vi "Describe Variant.vi"(11 "Variant":variant) -> (1 "Type Description":string, 2 "Description":string, 3 "Variant Description":string)   [LabVIEW 2020, in "Comparator.lvclass"]
uses:
  Comparator.lvclass
  <vilib>/Utility/Data Type/NI_Data Type.lvlib
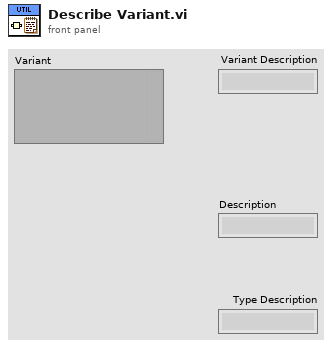
[diagram p1: front panel]
types:
  T1 = typedef "NI_Data Type.lvlib/Data Type.ctl" = enum8{"Invalid Type", "Void", "I8", "I16", "I32", "I64", "U8", "U16", "U32", "U64", "Single Float", "Double Float", "Extended Float", "Single Complex", "Double Complex", "Extended Complex", "Enum U8", "Enum U16", "Enum U32", "Enum U64", "Single Float With Unit", "Double Float With Unit", "Extended Float With Unit", "Single Complex with Unit", "Double Complex with Unit", "Extended Complex with Unit", "Boolean", "String", "Path", "Picture", "Tag", "Array", "Cluster", "Variant", "LV Variant", "Waveform", "Timestamp", "Digital Waveform", "Digital Data", "ExpressData", "Refnum", "External Data", "VI", "Poly VI", "LabVIEW Class Instance", "Fixed Point", "Set Collection", "Map Collection"}
  T2 = enum8{"Invalid Type", "Void", "I8", "I16", "I32", "I64", "U8", "U16", "U32", "U64", "Single Float", "Double Float", "Extended Float", "Single Complex", "Double Complex", "Extended Complex", "Enum U8", "Enum U16", "Enum U32", "Enum U64", "Single Float With Unit", "Double Float With Unit", "Extended Float With Unit", "Single Complex with Unit", "Double Complex with Unit", "Extended Complex with Unit", "Boolean", "String", "Path", "Picture", "Tag", "Array", "Cluster", "Variant", "LV Variant", "Waveform", "Timestamp", "Digital Waveform", "Digital Data", "ExpressData", "Refnum", "External Data", "VI", "Poly VI", "LabVIEW Class Instance", "Fixed Point", "Set Collection", "Map Collection"}
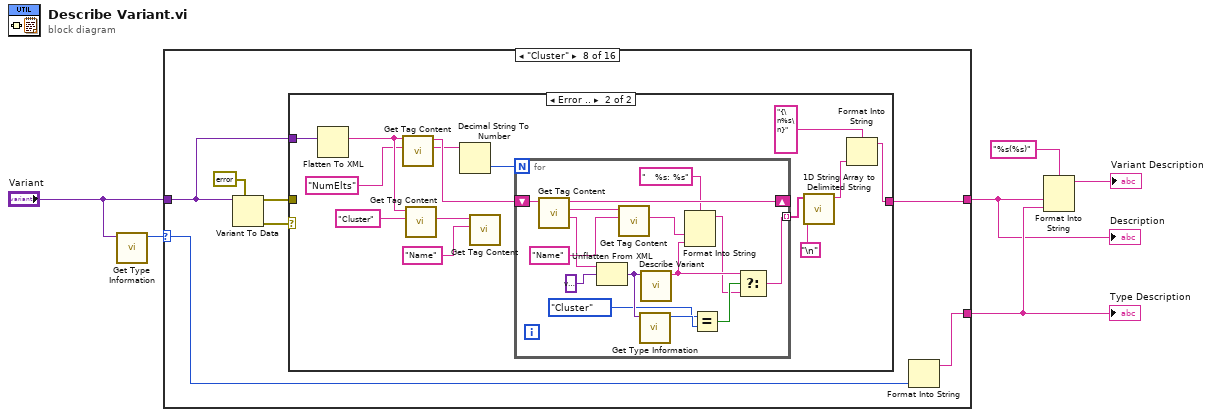
[diagram p0: block diagram]
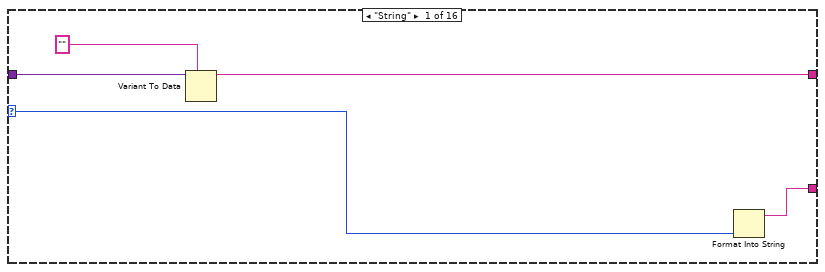
[diagram p2: hidden frame]
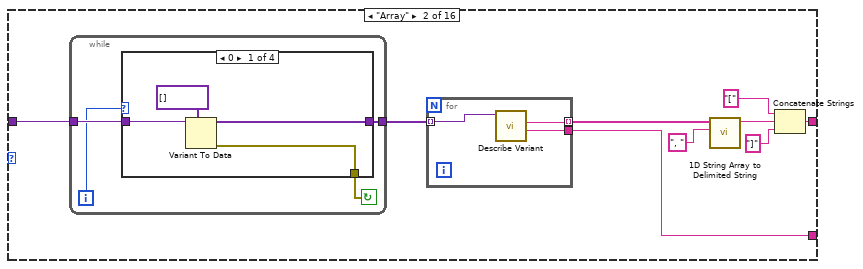
[diagram p3: hidden frame]
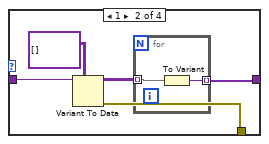
[diagram p4: hidden frame]
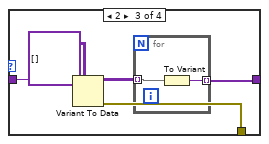
[diagram p5: hidden frame]
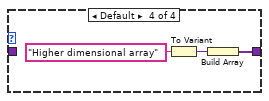
[diagram p6: hidden frame]
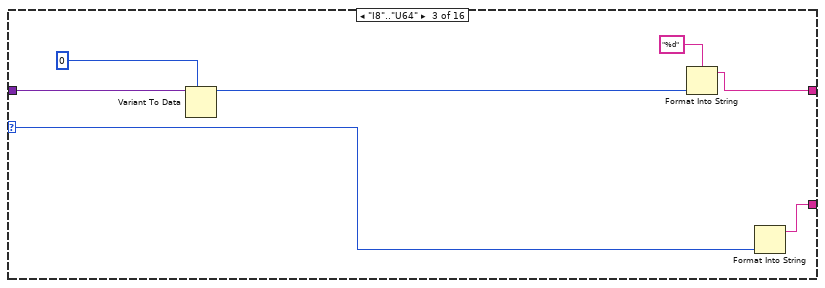
[diagram p7: hidden frame]
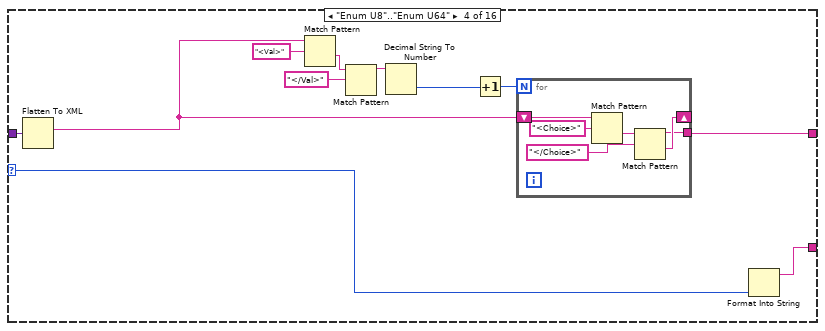
[diagram p8: hidden frame]
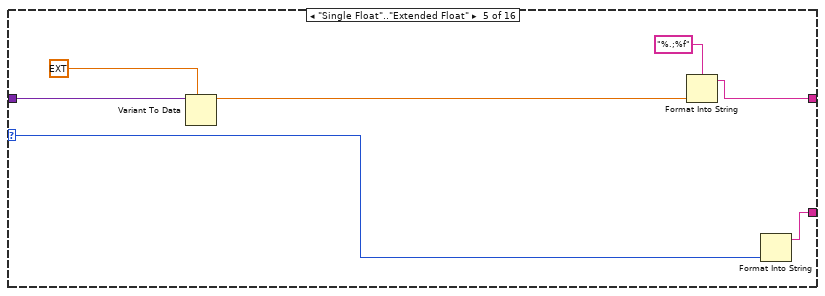
[diagram p9: hidden frame]
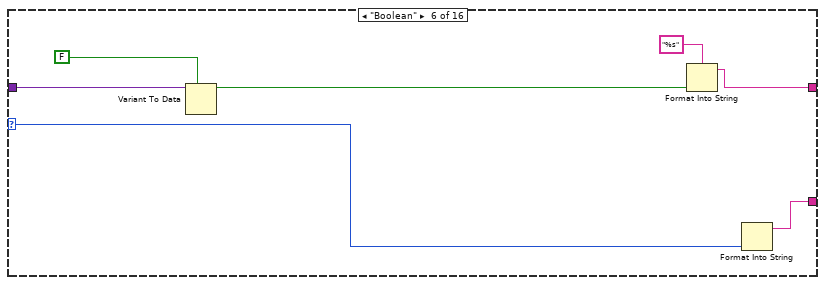
[diagram p10: hidden frame]
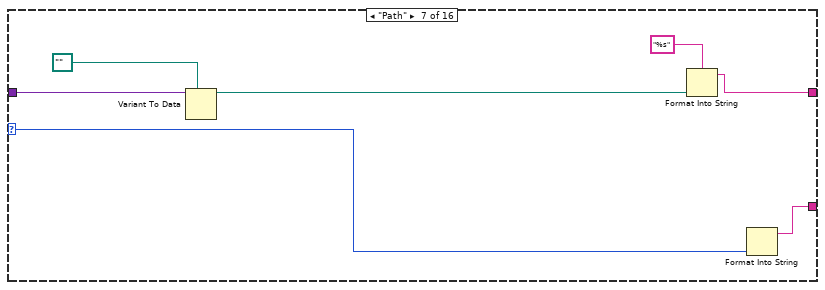
[diagram p11: hidden frame]
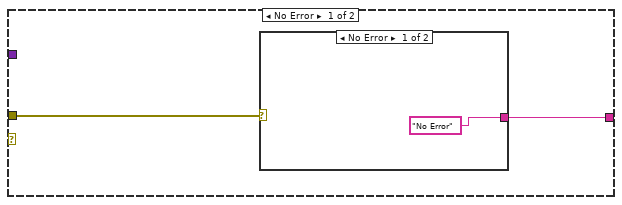
[diagram p12: hidden frame]
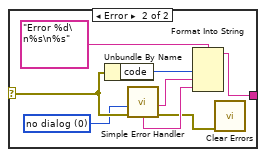
[diagram p13: hidden frame]
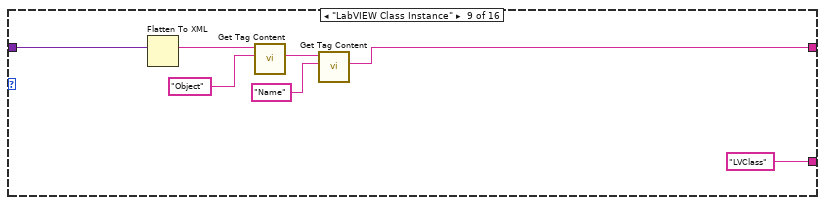
[diagram p14: hidden frame]
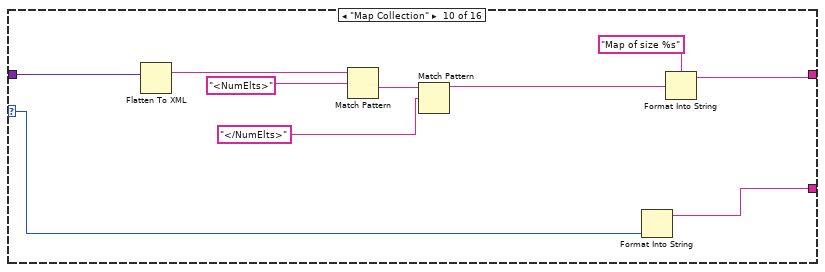
[diagram p15: hidden frame]
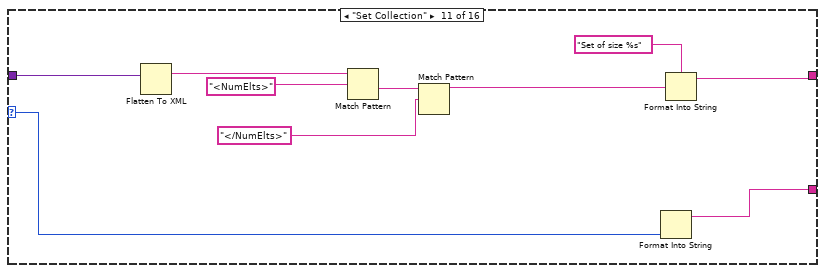
[diagram p16: hidden frame]
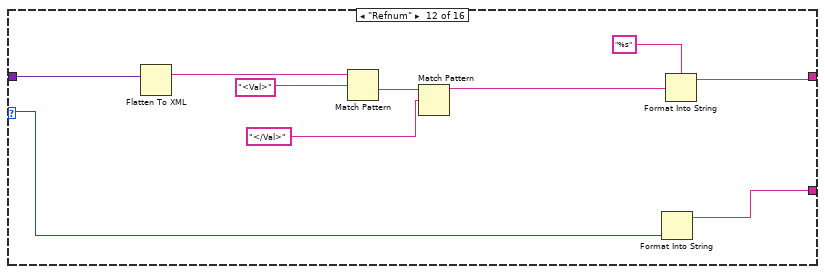
[diagram p17: hidden frame]
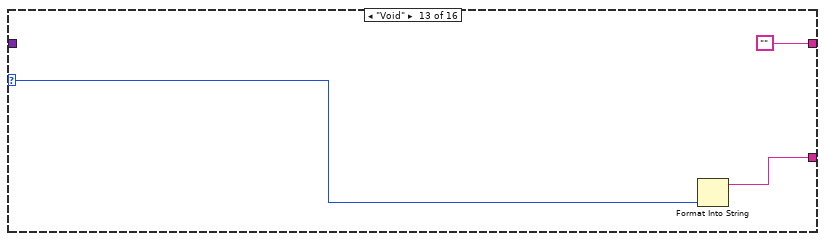
[diagram p18: hidden frame]
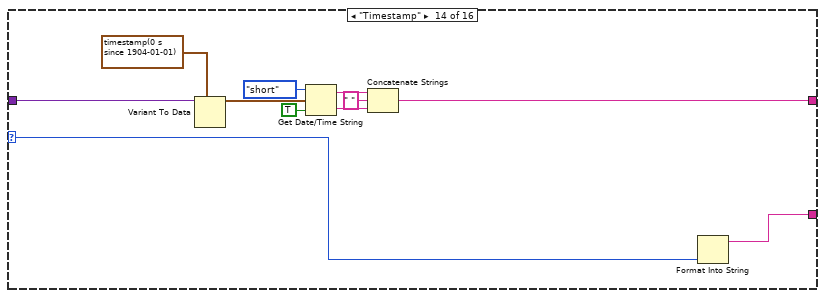
[diagram p19: hidden frame]
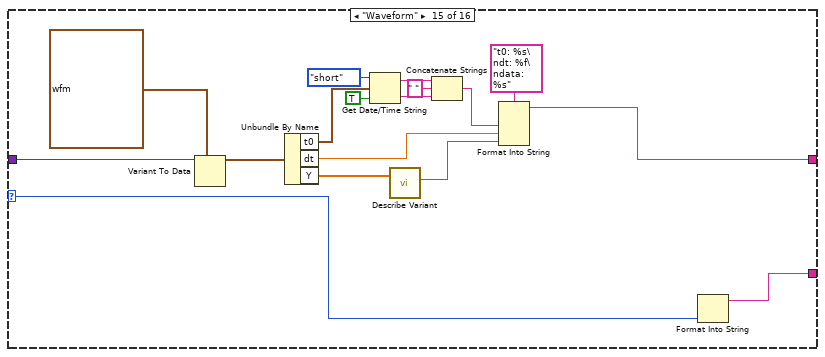
[diagram p20: hidden frame]
diagram:
  n1 = call <vilib>:"Get Type Information.vi"("variant"="Variant") -> ("type"=w5:T1)  [unwired: 6 in, 4 out]
  n2 = case shown="\"Cluster\"" w5 {
    selector: w5 -> [w7 _ w49 w65 w73 w80 w87 w98 _ w148 w158 w168 w180 w191 w208 w209]
    tunnel: "Variant" -> [w11 w20 w55 w57 w79 w86 w93 w94 w147 w157 w167 w177 _ w189 w206 w212]
    tunnel: [w10 w15 w51 w56 w75 w82 w89 w96 w141 w150 w160 w170 "" w181 w192 w211] -> w2
    tunnel: [w8 w12 w50 w66 w74 w81 w88 w97 "LVClass" w149 w159 w169 w179 w190 w207 w210] -> w4
    frame "String" {
      n3 = Variant To Data(type="", Variant=w11) -> (data=w10:string)  [unwired: 1 in, 1 out]
      n4 = Format Into String(w7) -> (resulting string=w8:string)  [unwired: 3 in, 1 out]
    }
    frame "Array" {
      n5 = while {
        tunnel: w20 -> [w24]
        tunnel: [w23] -> w19
        i -> [w22]
        stop <- w21 continue-if-true
        n6 = case shown="0" w22 {
          tunnel: w24 -> [w28 w33 w40 _]
          tunnel: [w26 w30 w37 w43] -> w23
          tunnel: [w25 w29 w36 _] -> w21
          frame 0 {
            n7 = Variant To Data(type=variant[] [], Variant=w28) -> (data=w26:variant[], error out=w25:errorcluster)  [unwired: 1 in]
          }
          frame 1 {
            n8 = Variant To Data(type=variant[][] [], Variant=w33) -> (data=w31:variant[][], error out=w29:errorcluster)  [unwired: 1 in]
            n9 = for {
              tunnel: w31 -> [w35] mode=indexing
              tunnel: [w34] -> w30 mode=indexing
              n10 = To Variant(anything=w35) -> (Variant=w34:variant)
            }
          }
          frame 2 {
            n11 = Variant To Data(type=variant[][][] [], Variant=w40) -> (data=w38:variant[][][], error out=w36:errorcluster)  [unwired: 1 in]
            n12 = for {
              tunnel: w38 -> [w42] mode=indexing
              tunnel: [w41] -> w37 mode=indexing
              n13 = To Variant(anything=w42) -> (Variant=w41:variant)
            }
          }
          frame Default {
            n14 = To Variant(anything="Higher dimensional array") -> (Variant=w44:variant)
            n15 = Build Array(w44) -> (w43:variant[])
          }
        }
      }
      n16 = for {
        tunnel: w19 -> [w48] mode=indexing
        tunnel: [w46] -> w17 mode=indexing
        tunnel: [w47] -> w12
        n17 = call "Describe Variant.vi"("Variant"=w48) -> ("Type Description"=w47:string, "Description"=w46:string)  [unwired: 8 in, 1 out]
      }
      n18 = call <vilib>:"1D String Array to Delimited String.vi"("delimiter"=", ", "string array"=w17) -> ("delimited string"=w16:string)  [unwired: 9 in]
      n19 = Concatenate Strings("[", w16, "]") -> (w15:string)
    }
    frame "I8".."U64" {
      n20 = Variant To Data(type=i64 0, Variant=w55) -> (data=w53:i64)  [unwired: 1 in, 1 out]
      n21 = Format Into String(format string="%d", w53) -> (resulting string=w51:string)  [unwired: 2 in, 1 out]
      n22 = Format Into String(w49) -> (resulting string=w50:string)  [unwired: 3 in, 1 out]
    }
    frame "Enum U8".."Enum U64" {
      n23 = Flatten To XML(6:w57) -> (2:w60:string)
      n24 = Match Pattern(string=w60, regular expression="<Val>" ("string")) -> (after substring=w61:string)  [unwired: 1 in, 3 out]
      n25 = Match Pattern(string=w61, regular expression="</Val>") -> (before substring=w62:string)  [unwired: 1 in, 3 out]
      n26 = Decimal String To Number(string=w62) -> (number=w63:i32)  [unwired: 2 in, 1 out]
      n27 = Increment(x=w63) -> (x+1=w64:i32)
      n28 = for {
        N: w64 -> [_]
        shift-right: [w68] -> _
        shift-left: w60 -> [w70]
        tunnel: [w67] -> w56
        n29 = Match Pattern(string=w70, regular expression="<Choice>" ("string")) -> (after substring=w72:string)  [unwired: 1 in, 3 out]
        n30 = Match Pattern(string=w72, regular expression="</Choice>") -> (before substring=w67:string, after substring=w68:string)  [unwired: 1 in, 2 out]
      }
      n31 = Format Into String(w65) -> (resulting string=w66:string)  [unwired: 3 in, 1 out]
    }
    frame "Single Float".."Extended Float" {
      n32 = Variant To Data(type=ext 0.0, Variant=w79) -> (data=w77:ext)  [unwired: 1 in, 1 out]
      n33 = Format Into String(format string="%.;%f", w77) -> (resulting string=w75:string)  [unwired: 2 in, 1 out]
      n34 = Format Into String(w73) -> (resulting string=w74:string)  [unwired: 3 in, 1 out]
    }
    frame "Boolean" {
      n35 = Variant To Data(type=FALSE, Variant=w86) -> (data=w84:bool)  [unwired: 1 in, 1 out]
      n36 = Format Into String(format string="%s", w84) -> (resulting string=w82:string)  [unwired: 2 in, 1 out]
      n37 = Format Into String(w80) -> (resulting string=w81:string)  [unwired: 3 in, 1 out]
    }
    frame "Path" {
      n38 = Variant To Data(type=path "", Variant=w93) -> (data=w91:path)  [unwired: 1 in, 1 out]
      n39 = Format Into String(format string="%s", w91) -> (resulting string=w89:string)  [unwired: 2 in, 1 out]
      n40 = Format Into String(w87) -> (resulting string=w88:string)  [unwired: 3 in, 1 out]
    }
    frame "Cluster" {
      n41 = Variant To Data(type=errorcluster {"status"=FALSE, "code"=0, "source"=""} ("error in"), Variant=w94) -> (data=w99:errorcluster, error out=w95:errorcluster)  [unwired: 1 in]
      n42 = case shown="Error .." w95 {
        tunnel: w99 -> [w102 _]
        tunnel: [w101 w112] -> w96
        tunnel: w94 -> [_ w125]
        frame No Error {
          n43 = case shown="No Error" w102 {
            selector: w102 -> [_ w108]
            tunnel: ["No Error" w110] -> w101
            frame No Error {
            }
            frame Error {
              w105 = u16 0 items=["no dialog", "OK message", "continue or stop message", "OK message + warnings", "continue/stop + warnings"] ("type of dialog (OK msg:1)")
              n44 = Unbundle By Name(w108) -> ("code"=w111:i32)
              n45 = call <vilib>:"Simple Error Handler.vi"("type of dialog (OK msg:1)"=w105, "error in (no error)"=w108) -> ("source out"=w107:string, "error out"=w104:errorcluster, "message"=w106:string)  [unwired: 3 in, 2 out]
              n46 = Format Into String(format string="Error %d\n%s\n%s", w111, w107, w106) -> (resulting string=w110:string)  [unwired: 2 in, 1 out]
              n47 = call <vilib>:"Clear Errors.vi"("error in (no error)"=w104) -> ()  [unwired: 5 in, 2 out]
            }
          }
        }
        frame Error {
          n48 = Flatten To XML(6:w125) -> (2:w120:string)
          n49 = call "Get Tag Content.vi"("Tag"="NumElts" ("regular expression"), "xml string in"=w120) -> ("Tag content"=w117:string, "After end of tag"=w118:string)  [unwired: 7 in, 1 out]
          n50 = call "Get Tag Content.vi"("Tag"="Cluster", "xml string in"=w120) -> ("Tag content"=w122:string)  [unwired: 7 in, 2 out]
          n51 = Decimal String To Number(string=w117) -> (number=w116:i32)  [unwired: 2 in, 1 out]
          n52 = call "Get Tag Content.vi"("Tag"="Name" ("regular expression"), "xml string in"=w122) -> ()  [unwired: 7 in, 3 out]
          n53 = for {
            N: w116 -> [_]
            tunnel: [w126] -> w123 mode=indexing
            shift-right: [w139] -> _
            shift-left: w118 -> [w140]
            n54 = call "Get Tag Content.vi"("xml string in"=w140) -> ("Tag with Content"=w133:string, "Tag content"=w136:string, "After end of tag"=w139:string)  [unwired: 8 in]
            n55 = Unflatten From XML(xml string=w133, type=variant) -> (value=w132:variant)  [unwired: 1 in, 1 out]
            n56 = call "Get Tag Content.vi"("Tag"="Name" ("regular expression"), "xml string in"=w136) -> ("Tag content"=w137:string)  [unwired: 7 in, 2 out]
            n57 = call <vilib>:"Get Type Information.vi"("variant"=w132) -> ("type"=w131:T1)  [unwired: 6 in, 4 out]
            n58 = call "Describe Variant.vi"("Variant"=w132) -> ("Variant Description"=w128:string)  [unwired: 8 in, 2 out]
            n59 = Format Into String(format string="   %s: %s", w137, w128) -> (resulting string=w127:string)  [unwired: 2 in, 1 out]
            n60 = Equal?(x=T2."Cluster", y=w131) -> (x = y?=w129:bool)
            n61 = Select(t=w128, s=w129, f=w127) -> (s? t:f=w126:string)
          }
          n62 = call <vilib>:"1D String Array to Delimited String.vi"("delimiter"="\n", "string array"=w123) -> ("delimited string"=w113:string)  [unwired: 9 in]
          n63 = Format Into String(format string="{\n%s\n}", w113) -> (resulting string=w112:string)  [unwired: 2 in, 1 out]
        }
      }
      n64 = Format Into String(w98) -> (resulting string=w97:string)  [unwired: 3 in, 1 out]
    }
    frame "LabVIEW Class Instance" {
      n65 = Flatten To XML(6:w147) -> (2:w143:string)
      n66 = call "Get Tag Content.vi"("Tag"="Object", "xml string in"=w143) -> ("Tag content"=w145:string)  [unwired: 7 in, 2 out]
      n67 = call "Get Tag Content.vi"("Tag"="Name" ("regular expression"), "xml string in"=w145) -> ("Tag content"=w141:string)  [unwired: 7 in, 2 out]
    }
    frame "Map Collection" {
      n68 = Flatten To XML(6:w157) -> (2:w152:string)
      n69 = Match Pattern(string=w152, regular expression="<NumElts>" ("string")) -> (after substring=w155:string)  [unwired: 1 in, 3 out]
      n70 = Match Pattern(string=w155, regular expression="</NumElts>" ("string")) -> (before substring=w153:string)  [unwired: 1 in, 3 out]
      n71 = Format Into String(w148) -> (resulting string=w149:string)  [unwired: 3 in, 1 out]
      n72 = Format Into String(format string="Map of size %s", w153) -> (resulting string=w150:string)  [unwired: 2 in, 1 out]
    }
    frame "Set Collection" {
      n73 = Flatten To XML(6:w167) -> (2:w162:string)
      n74 = Match Pattern(string=w162, regular expression="<NumElts>" ("string")) -> (after substring=w165:string)  [unwired: 1 in, 3 out]
      n75 = Match Pattern(string=w165, regular expression="</NumElts>" ("string")) -> (before substring=w163:string)  [unwired: 1 in, 3 out]
      n76 = Format Into String(w158) -> (resulting string=w159:string)  [unwired: 3 in, 1 out]
      n77 = Format Into String(format string="Set of size %s", w163) -> (resulting string=w160:string)  [unwired: 2 in, 1 out]
    }
    frame "Refnum" {
      n78 = Flatten To XML(6:w177) -> (2:w172:string)
      n79 = Match Pattern(string=w172, regular expression="<Val>" ("string")) -> (after substring=w175:string)  [unwired: 1 in, 3 out]
      n80 = Match Pattern(string=w175, regular expression="</Val>" ("string")) -> (before substring=w173:string)  [unwired: 1 in, 3 out]
      n81 = Format Into String(w168) -> (resulting string=w169:string)  [unwired: 3 in, 1 out]
      n82 = Format Into String(format string="%s", w173) -> (resulting string=w170:string)  [unwired: 2 in, 1 out]
    }
    frame "Void" {
      n83 = Format Into String(w180) -> (resulting string=w179:string)  [unwired: 3 in, 1 out]
    }
    frame "Timestamp" {
      n84 = Variant To Data(type=timestamp(0 s since 1904-01-01) ("current time"), Variant=w189) -> (data=w187:timestamp)  [unwired: 1 in, 1 out]
      n85 = Get Date/Time String(date format (0)=enum16{"short", "long", "abbreviated"}."short", seconds (now)=w187, want seconds? (F)=TRUE) -> (date string=w184:string, time string=w183:string)
      n86 = Concatenate Strings(w184, " " ("string"), w183) -> (w181:string)
      n87 = Format Into String(w191) -> (resulting string=w190:string)  [unwired: 3 in, 1 out]
    }
    frame "Waveform" {
      n88 = Variant To Data(type=waveform(dbl) {"t0"=timestamp(0 s since 1904-01-01), "dt"=1.0, "Y"=[]} ("Waveform"), Variant=w206) -> (data=w199:waveform(dbl))  [unwired: 1 in, 1 out]
      n89 = Unbundle By Name(w199) -> ("t0"=w198:timestamp, "dt"=w195:dbl, "Y"=w194:dbl[])
      n90 = Get Date/Time String(date format (0)=enum16{"short", "long", "abbreviated"}."short", seconds (now)=w198, want seconds? (F)=TRUE) -> (date string=w202:string, time string=w201:string)
      n91 = call "Describe Variant.vi"("Variant"=w194) -> ("Description"=w193:string)  [unwired: 8 in, 2 out]
      n92 = Concatenate Strings(w202, " " ("string"), w201) -> (w197:string)
      n93 = Format Into String(format string="t0: %s\ndt: %f\ndata: %s", w197, w195, w193) -> (resulting string=w192:string)  [unwired: 2 in, 1 out]
      n94 = Format Into String(w208) -> (resulting string=w207:string)  [unwired: 3 in, 1 out]
    }
    frame Default {
      n95 = Flatten To XML(6:w212) -> (2:w211:string)
      n96 = Format Into String(w209) -> (resulting string=w210:string)  [unwired: 3 in, 1 out]
    }
  }
  "Type Description" <- w4
  "Description" <- w2
  n97 = Format Into String(format string="%s(%s)", w2, w4) -> (resulting string=→"Variant Description":string)  [unwired: 2 in, 1 out]
